vi "PSHet_DAQInAndOut.vi"() -> ()   [LabVIEW 2022 SP3]
uses:
  PSHet_DAQInAndOut_control.ctl
  <vilib>/DAQmx/read.llb/DAQmx Read (Analog 2D DBL NChan NSamp).vi
  <vilib>/Analysis/baseanly.llb/Mean (DBL).vi
  <vilib>/DAQmx/write.llb/DAQmx Write (Analog 1D DBL NChan 1Samp).vi
  <vilib>/DAQmx/create/channels.llb/DAQmx Create Channel (AI-Voltage-Basic).vi
  <vilib>/DAQmx/configure/timing.llb/DAQmx Timing (Sample Clock).vi
  <vilib>/DAQmx/create/channels.llb/DAQmx Create Channel (AO-Voltage-Basic).vi
  <vilib>/DAQmx/miscellaneous.llb/DAQmx Fill In Error Info.vi
  <vilib>/Analysis/NI_AALBase.lvlib
panel:
  in  "Phase offset (rad)":dbl
  out "Phase (1 = pi radians)":dbl(graph)=0.5644736182326506
  out "Amplitude / Re / Im":T1(graph)={"[0]"=0.015751873474111572, "[1]"=-0.0031687681651577076, "[2]"=0.015429855030424067, "[3]"=0.0, "[4]"=0.0, "[5]"=0.0, "[6]"=0.0, "[7]"=0.0, "[8]"=0.0}
  out "Samples per loop":i32=100
  in  "Channels to output":tag="Dev1/ao0:1"
  out "Iteration":i32=66065
  out "DAQ input error":errorcluster
  out "Output Phase (rad)":dbl=1.7733461721849446
  out "Output Amplitude":dbl=0.015751873474111572
  out "Status":string="Running PSHet..."
  in  "PAUSE":bool
  in  "Amplify amplitude by":dbl=1.0
  in  "DAQ Output range (V)":dbl=10.0
  in  "DAQ Input range (V)":dbl=10.0
  in  "Time per acquisiton (ms)":dbl=1.0
  in  "Sampling rate":dbl=100000.0
  in  "Channels to read":tag="Dev1/ai4:7"
  in  "stop":bool
  out "DAQ output error":errorcluster
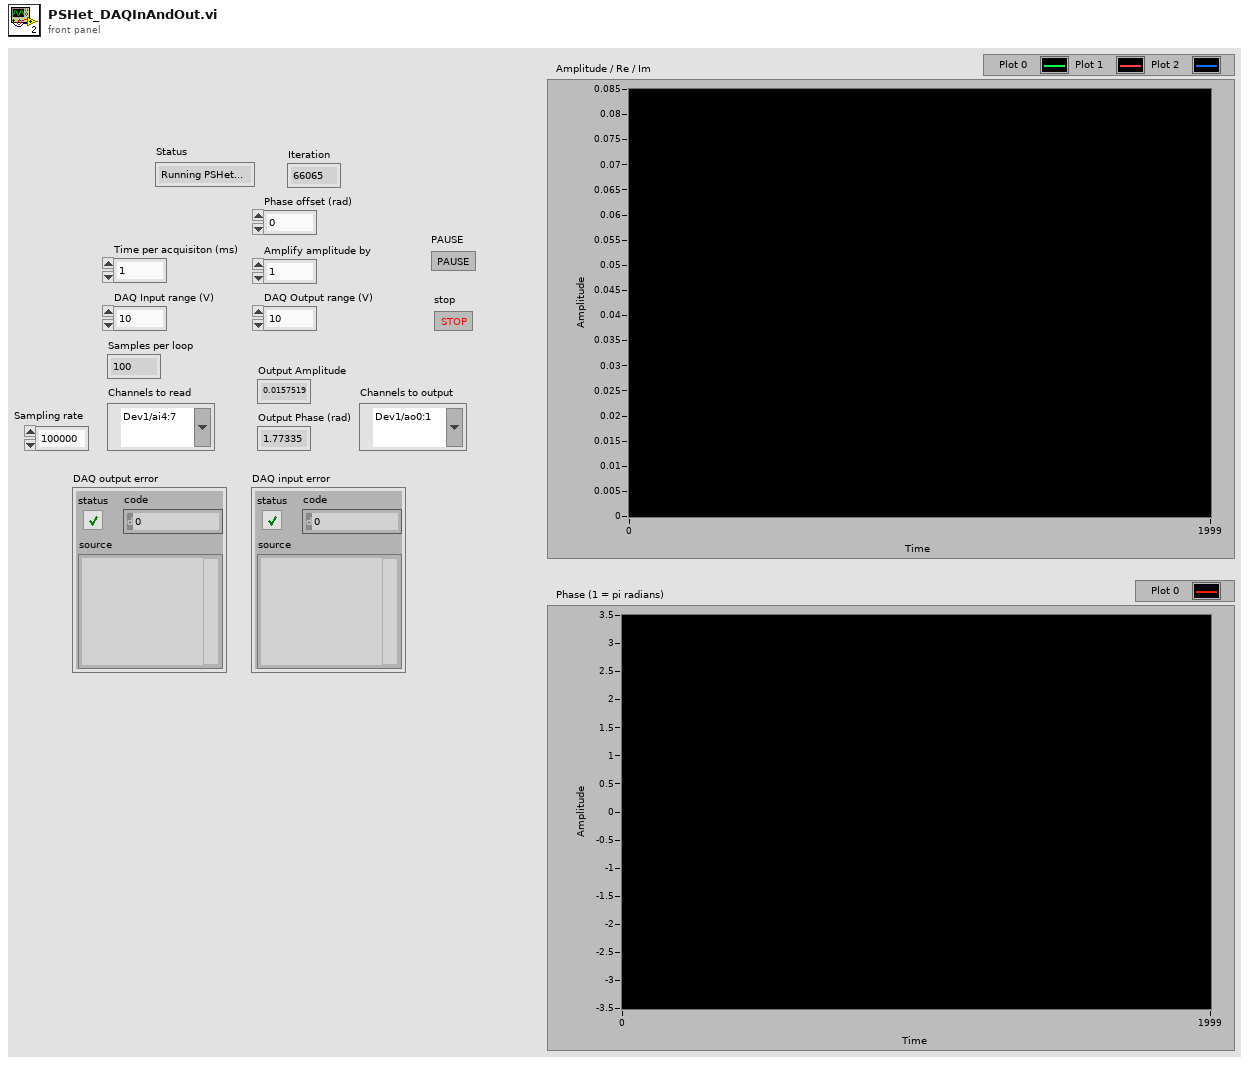
[diagram p1: front panel]
types:
  T1 = cluster{"[0]":dbl, "[1]":dbl, "[2]":dbl, "[3]":dbl, "[4]":dbl, "[5]":dbl, "[6]":dbl, "[7]":dbl, "[8]":dbl}
  T2 = typedef "PSHet_DAQInAndOut_control.ctl" = enum16{"Prepare DAQ task", "Run DAQ task", "Pause", "Close DAQ task"}
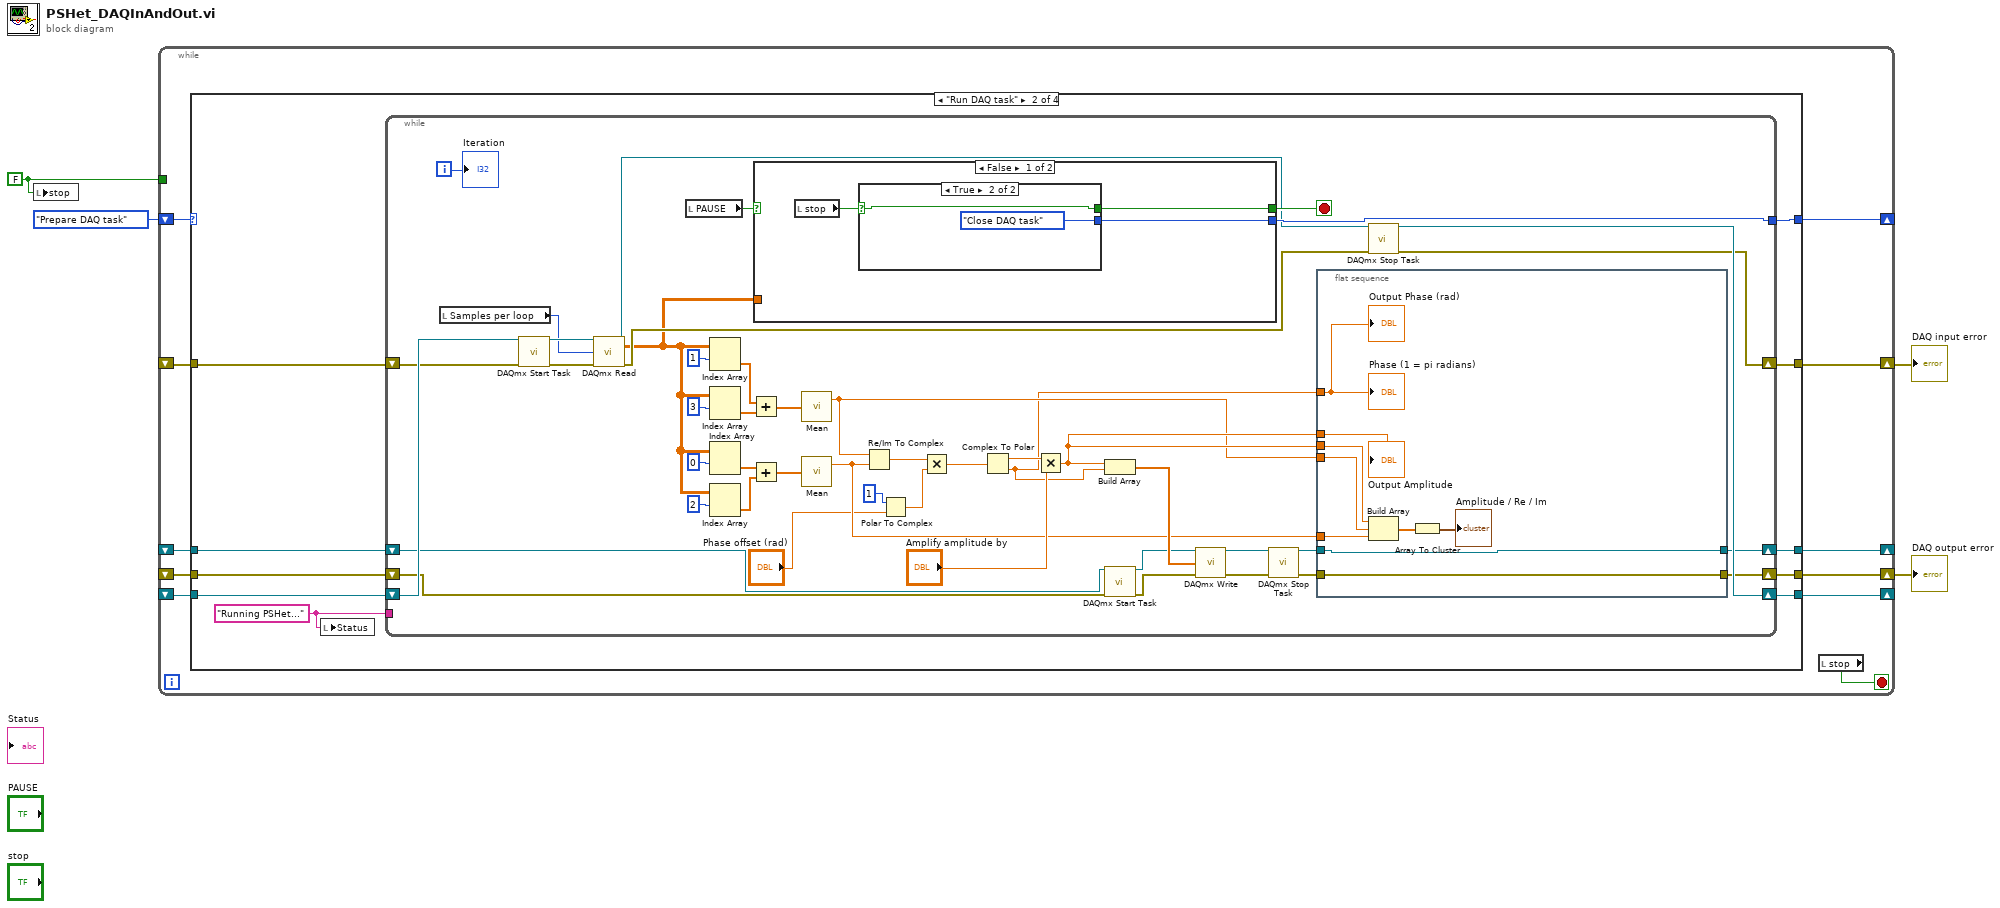
[diagram p0: block diagram]
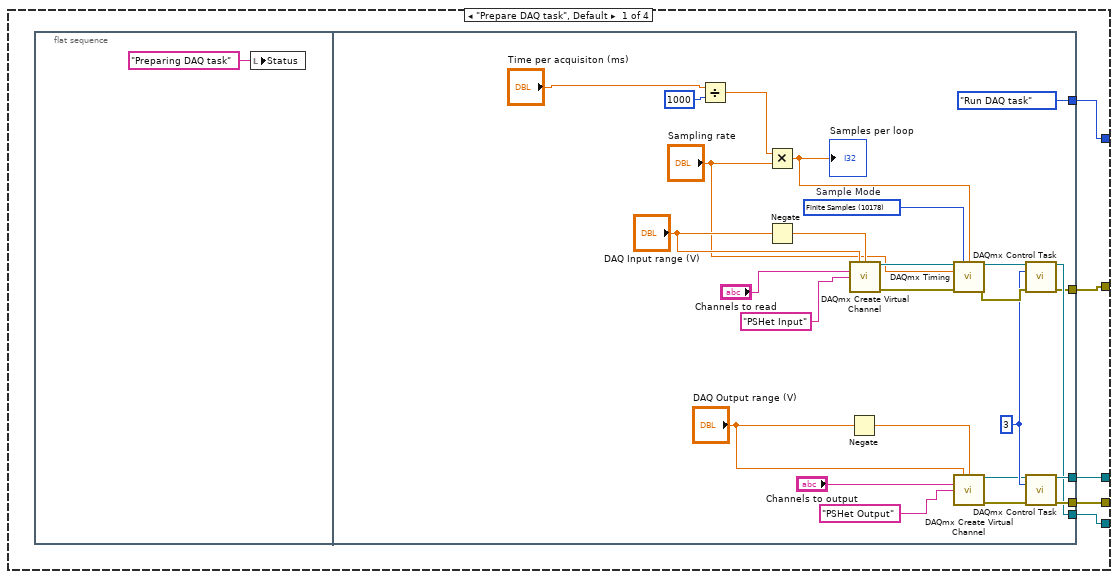
[diagram p2: hidden frame]
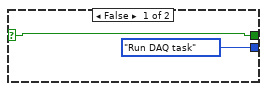
[diagram p3: hidden frame]
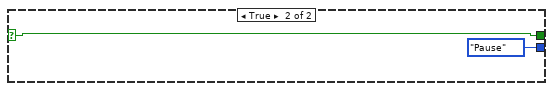
[diagram p4: hidden frame]
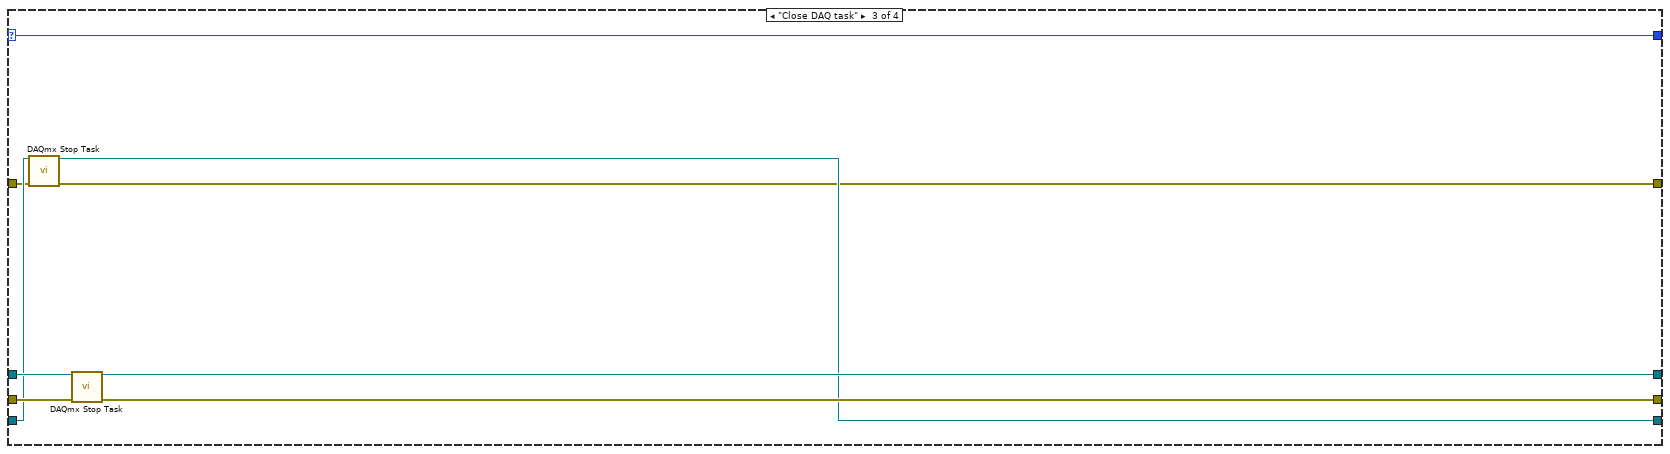
[diagram p5: hidden frame]
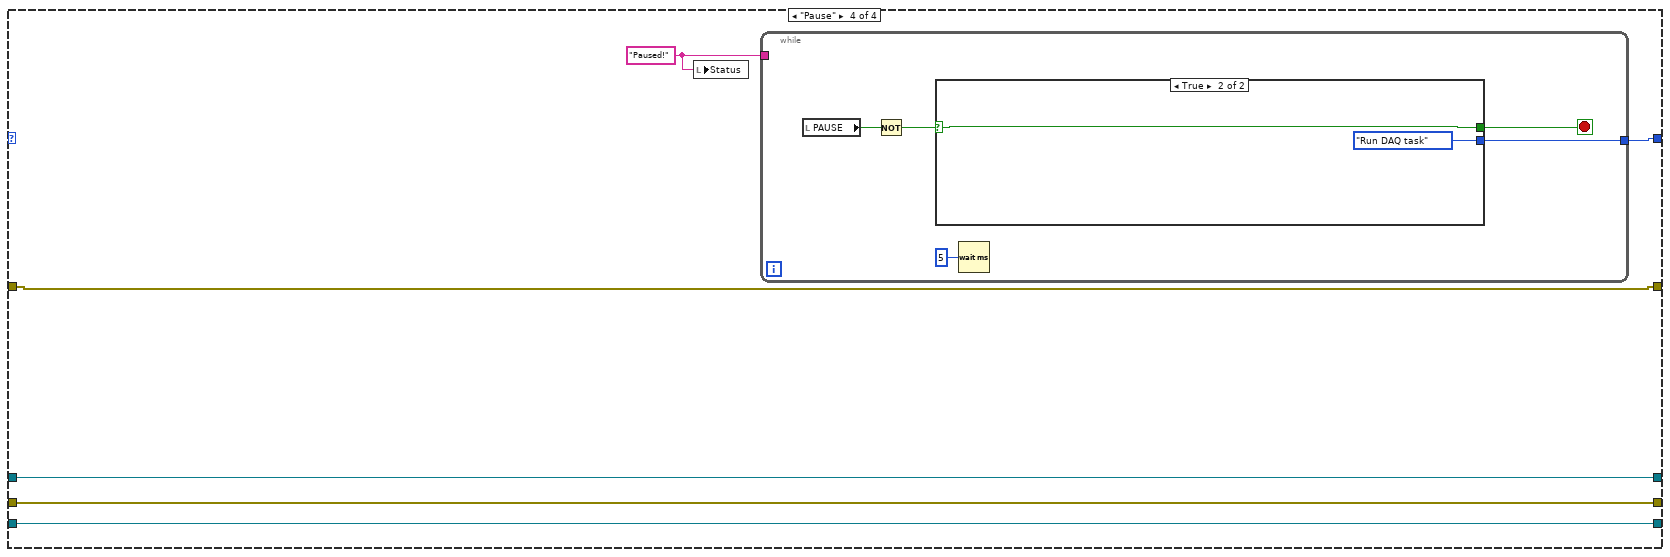
[diagram p6: hidden frame]
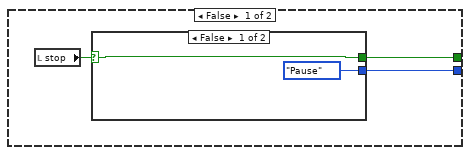
[diagram p7: hidden frame]
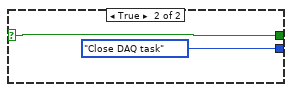
[diagram p8: hidden frame]
diagram:
  w1 = FALSE
  n1 = local write "stop"(w1) -> ()
  n2 = while {
    shift-right: [w14] -> _
    shift-left: _ -> [w6]
    shift-right: [w13] -> w2
    shift-left: _ -> [w5]
    shift-right: [w12] -> _
    shift-left: _ -> [w8]
    shift-right: [w11] -> w3
    shift-left: _ -> [w7]
    shift-right: [w10] -> _
    shift-left: PSHet_DAQInAndOut_control."Prepare DAQ task" -> [w15]
    tunnel: w1 -> [_]
    stop <- w9 stop-if-true
    n3 = case shown="\"Run DAQ task\"" w15 {
      selector: w15 -> [_ _ w122 _]
      tunnel: [w19 w50 w128 w134] -> w12
      tunnel: [w18 w51 w127 w133] -> w11
      tunnel: [w17 w53 w124 w132] -> w14
      tunnel: [w16 w52 w123 w131] -> w13
      tunnel: [w20 w49 w122 w135] -> w10
      tunnel: w8 -> [_ w57 w130 w134]
      tunnel: w7 -> [_ w56 w129 w133]
      tunnel: w6 -> [_ w55 w126 w132]
      tunnel: w5 -> [_ w54 w125 w131]
      frame "Prepare DAQ task", Default {
        n4 = flat-sequence {
          tunnel: [PSHet_DAQInAndOut_control."Run DAQ task"] -> w20
          tunnel: [w33] -> w19
          tunnel: [w32] -> w18
          tunnel: [w31] -> w17
          tunnel: [w30] -> w16
          frame #0 {
            n5 = local write "Status"("Preparing DAQ task") -> ()
          }
          frame #1 {
            w38 = 3
            w37 = 10178 items=["Finite Samples"=10178, "Continuous Samples"=10123, "Hardware Timed Single Point"=12522]  # Sample Mode
            n6 = Divide(x="Time per acquisiton (ms)", y=1000) -> (x/y=w24:dbl)
            n7 = Multiply(x=w24, y="Sampling rate") -> (x*y=w27:dbl)
            "Samples per loop" <- w27
            n8 = Negate(x="DAQ Input range (V)") -> (-x=w41:dbl)
            n9 = Negate(x="DAQ Output range (V)") -> (-x=w47:dbl)
            n10 = call-poly <vilib>:"DAQmx Create Virtual Channel.vi"("maximum value"="DAQ Input range (V)", "minimum value"=w41, "physical channels"="Channels to read", "name to assign"="PSHet Input") -> ("task out"=w40:refnum<k21>, "error out"=w39:errorcluster)  [unwired: 10 in]
            n11 = call-poly <vilib>:"DAQmx Timing.vi"("task/channels in"=w40, "sample mode"=w37, "samples per channel"=w27, "rate"="Sampling rate", "error in"=w39) -> ("task out"=w44:refnum<k21>, "error out"=w45:errorcluster)  [unwired: 9 in]
            n12 = call-poly <vilib>:"DAQmx Create Virtual Channel.vi"("maximum value"="DAQ Output range (V)", "minimum value"=w47, "physical channels"="Channels to output", "name to assign"="PSHet Output") -> ("task out"=w23:refnum<k21>, "error out"=w22:errorcluster)  [unwired: 10 in]
            n13 = call <vilib>:"DAQmx Control Task.vi"("task/channels in"=w44, "action"=w38, "error in"=w45) -> ("task out"=w31:refnum<k21>, "error out"=w30:errorcluster)  [unwired: 11 in]
            n14 = call <vilib>:"DAQmx Control Task.vi"("task/channels in"=w23, "action"=w38, "error in"=w22) -> ("task out"=w33:refnum<k21>, "error out"=w32:errorcluster)  [unwired: 11 in]
          }
        }
      }
      frame "Run DAQ task" {
        w48 = "Running PSHet..."
        n15 = local write "Status"(w48) -> ()
        n16 = while {
          shift-right: [w70] -> w50
          shift-left: w57 -> [w79]
          shift-right: [w68] -> w51
          shift-left: w56 -> [w78]
          shift-right: [w83] -> w53
          shift-left: w55 -> [w87]
          shift-right: [w82] -> w52
          shift-left: w54 -> [w85]
          tunnel: [w91] -> w49
          tunnel: w48 -> [_]
          i -> [w73]
          stop <- w90 stop-if-true
          n17 = local read "Samples per loop"() -> (w72:i32)
          n18 = call <vilib>:"DAQmx Start Task.vi"("task/channels in"=w87, "error in"=w85) -> ("task out"=w86:refnum<k21>, "error out"=w84:errorcluster)  [unwired: 12 in]
          n19 = call-poly <vilib>:"DAQmx Read.vi"("task/channels in"=w86, "number of samples per channel"=w72, "error in"=w84) -> ("task out"=w81:refnum<k21>, "data"=w66:dbl[][], "error out"=w80:errorcluster)  [unwired: 10 in]
          n20 = local read "PAUSE"() -> (w92:bool)
          n21 = Index Array(array=w66, index (row)=1) -> (element=w101:dbl[])  [unwired: 1 in]
          n22 = Index Array(array=w66, index (row)=3) -> (element=w100:dbl[])  [unwired: 1 in]
          n23 = Index Array(array=w66, index (row)=0) -> (element=w96:dbl[])  [unwired: 1 in]
          n24 = Index Array(array=w66, index (row)=2) -> (element=w95:dbl[])  [unwired: 1 in]
          n25 = Add(x=w101, y=w100) -> (x+y=w99:dbl[])
          n26 = Add(x=w96, y=w95) -> (x+y=w94:dbl[])
          n27 = case shown="False" w92 {
            selector: w92 -> [_ w121]
            tunnel: [w113 w121] -> w90
            tunnel: [w114 PSHet_DAQInAndOut_control."Pause"] -> w91
            tunnel: w66 -> [_ _]
            frame False {
              n28 = local read "stop"() -> (w115:bool)
              n29 = case shown="True" w115 {
                selector: w115 -> [w116 w118]
                tunnel: [PSHet_DAQInAndOut_control."Run DAQ task" PSHet_DAQInAndOut_control."Close DAQ task"] -> w114
                tunnel: [w116 w118] -> w113
                frame False {
                }
                frame True {
                }
              }
            }
            frame True {
            }
          }
          n30 = call-poly <vilib>:"Mean.vi"("X"=w99) -> ("mean"=w65:dbl)  [unwired: 1 out]
          n31 = call-poly <vilib>:"Mean.vi"("X"=w94) -> ("mean"=w64:dbl)  [unwired: 1 out]
          n32 = Re/Im To Complex(1:w64, 2:w65) -> (0:w60:cdb)
          n33 = Polar To Complex(1:"Phase offset (rad)", 2:1) -> (0:w58:cdb)
          n34 = Multiply(x=w60, y=w58) -> (x*y=w59:cdb)
          n35 = Complex To Polar(r * e^(i*theta)=w59) -> (r=w89:dbl, theta=w63:dbl)
          n36 = Multiply(x=w89, y="Amplify amplitude by") -> (x*y=w67:dbl)
          n37 = Build Array(w67, w63) -> (w93:dbl[])
          n38 = call <vilib>:"DAQmx Start Task.vi"("task/channels in"=w79, "error in"=w78) -> ("task out"=w77:refnum<k21>, "error out"=w76:errorcluster)  [unwired: 12 in]
          n39 = call-poly <vilib>:"DAQmx Write.vi"("task/channels in"=w77, "data"=w93, "error in"=w76) -> ("task out"=w75:refnum<k21>, "error out"=w74:errorcluster)  [unwired: 10 in, 1 out]
          n40 = call <vilib>:"DAQmx Stop Task.vi"("task/channels in"=w75, "error in"=w74) -> ("task out"=w71:refnum<k21>, "error out"=w69:errorcluster)  [unwired: 12 in]
          n41 = flat-sequence {
            tunnel: w67 -> [w108]
            tunnel: w71 -> [w112]
            tunnel: [w112] -> w70
            tunnel: w69 -> [w111]
            tunnel: [w111] -> w68
            tunnel: w67 -> [w110]
            tunnel: w63 -> [w104]
            tunnel: w65 -> [w106]
            tunnel: w64 -> [w105]
            frame #0 {
              n42 = Build Array(w108, w106, w105) -> (w109:dbl[])
              n43 = Array To Cluster(array=w109) -> (cluster=→"Amplitude / Re / Im":T1)
              "Phase (1 = pi radians)" <- w104
              "Output Amplitude" <- w110
              "Output Phase (rad)" <- w104
            }
          }
          n44 = call <vilib>:"DAQmx Stop Task.vi"("task/channels in"=w81, "error in"=w80) -> ("task out"=w83:refnum<k21>, "error out"=w82:errorcluster)  [unwired: 12 in]
          "Iteration" <- w73
        }
      }
      frame "Close DAQ task" {
        n45 = call <vilib>:"DAQmx Stop Task.vi"("task/channels in"=w126, "error in"=w125) -> ("task out"=w124:refnum<k21>, "error out"=w123:errorcluster)  [unwired: 12 in]
        n46 = call <vilib>:"DAQmx Stop Task.vi"("task/channels in"=w130, "error in"=w129) -> ("task out"=w128:refnum<k21>, "error out"=w127:errorcluster)  [unwired: 12 in]
      }
      frame "Pause" {
        w136 = "Paused!"
        n47 = local write "Status"(w136) -> ()
        n48 = while {
          tunnel: w136 -> [_]
          tunnel: [w140] -> w135
          stop <- w139 stop-if-true
          n49 = local read "PAUSE"() -> (w138:bool)
          n50 = Not(x=w138) -> (.not. x?=w137:bool)
          n51 = case shown="True" w137 {
            selector: w137 -> [_ w150]
            tunnel: [w142 w150] -> w139
            tunnel: [w143 PSHet_DAQInAndOut_control."Run DAQ task"] -> w140
            frame False {
              n52 = local read "stop"() -> (w144:bool)
              n53 = case shown="False" w144 {
                selector: w144 -> [w145 w147]
                tunnel: [PSHet_DAQInAndOut_control."Pause" PSHet_DAQInAndOut_control."Close DAQ task"] -> w143
                tunnel: [w145 w147] -> w142
                frame False {
                }
                frame True {
                }
              }
            }
            frame True {
            }
          }
          n54 = Wait (ms)(milliseconds to wait=5) -> ()  [unwired: 1 out]
        }
      }
    }
    n55 = local read "stop"() -> (w9:bool)
  }
  "DAQ output error" <- w3
  "DAQ input error" <- w2
